vi "write_synch_op.vi"(11 "Bus":T1) -> ()   [LabVIEW 2011]
uses:
  Common/demux_command.ctl
  <vilib>/rvi/DataTransferAndStorage/Container/Common/niFpgaContainerExecOnDevCompGetState.vi
  <vilib>/rvi/FIFO/Fifo_Resource/nirvififoEmulationSetSize.vi
  <vilib>/rvi/DataTransferAndStorage/Container/Common/niFpgaContainerGetUniqueNameForEmu.vi
  <vilib>/rvi/interface/RandomDataEmulation/nirviRandomDataFPGAFIFO.vi
  <vilib>/rvi/interface/RandomDataEmulation/niFpgaRandomDataHandleErrors.vi
  <vilib>/rvi/eio/common/nirviEmuReportErrorAndStop.vi
  <vilib>/rvi/DataTransferAndStorage/Container/XNode/niFpgaContainer.xnode
  <vilib>/rvi/FIFO/Fifo_Resource/niFpgaFifoEmulationRefIn.vi
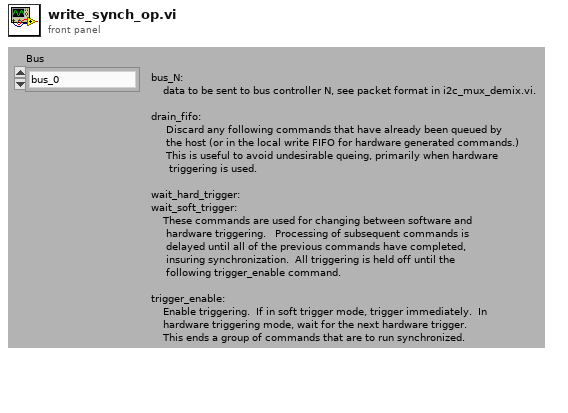
[diagram p1: front panel]
types:
  T1 = typedef "demux_command.ctl" = enum8{"bus_0", "bus_1", "bus_2", "invalid_3", "invalid_4", "drain_fifo", "wait_hard_trigger", "wait_soft_trigger", "trigger_enable"}
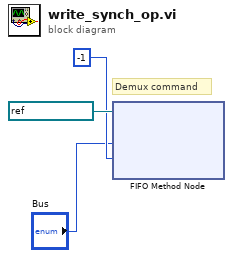
[diagram p0: block diagram]
diagram:
  # "Demux command"
  n1 = xnode ("FIFO Method Node")("Element"="Bus", "Timeout"=-1, "FIFO In"=refnum<k21> "Local write" ("FIFO")) -> ()  [unwired: 2 out]
